vi "CB Local Sense Test_v2.vi"(8 "error in (no error)":errorcluster, 11 "Control Board VISA":refnum<visa-resource-name>) -> (0 "error out":errorcluster, 2 "MSE Array":dbl[](array[numeric]), 3 "Pass?":bool)   [LabVIEW 2022 SP3]
panel:
  out "Voltage Readings":dbl[][](array[numeric])
  out "Message OUT":string
  in  "Message IN":string
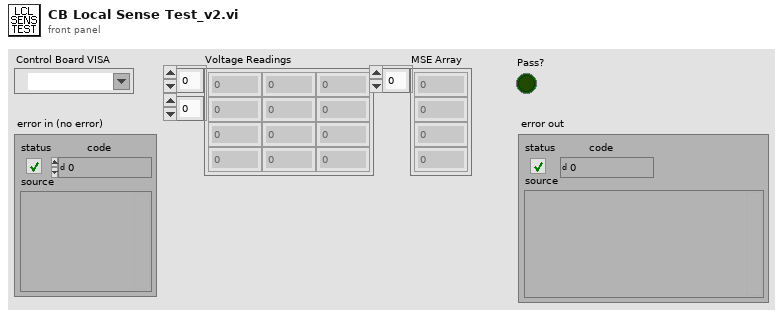
[diagram p1: front panel]
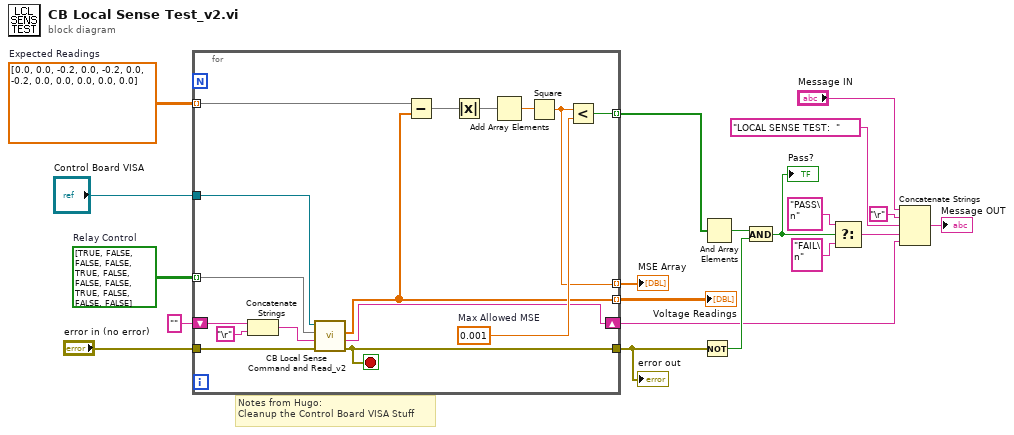
[diagram p0: block diagram]
diagram:
  w1 = dbl[][] [[0.0, 0.0, -0.2], [0.0, -0.2, 0.0], [-0.2, 0.0, 0.0], [0.0, 0.0, 0.0]]  # Expected Readings
  w19 = bool[][] [[TRUE, FALSE, FALSE], [FALSE, TRUE, FALSE], [FALSE, FALSE, TRUE], [FALSE, FALSE, FALSE]]  # Relay Control
  # "Notes from Hugo:\nCleanup the Control Board VISA Stuff"
  n1 = for {
    tunnel: [w35] -> w16
    tunnel: "error in (no error)" -> [w36]
    tunnel: w1 -> [w32] mode=indexing
    tunnel: [w29] -> w20 mode=indexing
    tunnel: w19 -> [w28] mode=indexing
    tunnel: [w27] -> w15 mode=indexing
    tunnel: [w26] -> w14 mode=indexing
    shift-right: [w25] -> w7
    shift-left: "" -> [w24]
    tunnel: "Control Board VISA" -> [w21]
    stop <- w35 stop-if-true
    w30 = 0.001  # Max Allowed MSE
    n2 = Concatenate Strings(w24, "\r") -> (w23:string)
    n3 = call "CB Local Sense Command and Read_v2.vi"("error in (no error)"=w36, "Message IN"=w23, "Relay Control"=w28, "Control Board VISA"=w21) -> ("error out"=w35:errorcluster, "Message OUT"=w25:string, "Voltage Array"=w27:dbl[])  [unwired: 4 in, 1 out]
    n4 = Subtract(x=w32, y=w27) -> (x-y=w34:dbl[])
    n5 = Absolute Value(x=w34) -> (abs(x)=w33:dbl[])
    n6 = Add Array Elements(numeric array=w33) -> (sum=w31:dbl)
    n7 = Square(x=w31) -> (x^2=w26:dbl)
    n8 = Less?(x=w26, y=w30) -> (x < y?=w29:bool)
  }
  "error out" <- w16
  "Voltage Readings" <- w15
  "MSE Array" <- w14
  n9 = Not(x=w16) -> (.not. x?=w17:bool)
  n10 = And Array Elements(Boolean array=w20) -> (logical AND=w18:bool)
  n11 = And(x=w18, y=w17) -> (x .and. y?=w9:bool)
  "Pass?" <- w9
  n12 = Select(t="PASS\n", s=w9, f="FAIL\n") -> (s? t:f=w8:string)
  n13 = Concatenate Strings("Message IN", "\r", "LOCAL SENSE TEST:  ", w8, w7) -> (→"Message OUT":string)
